vi "Adapt Experimental Data to Graph Entry.vi"(1 "Experiment Data":T1, 2 "Load Path":path) -> (0 "Populated Entry":T2)   [LabVIEW 2013]
uses:
  Serialization/Experiment/1.0.0/Types/Experiment Data.ctl
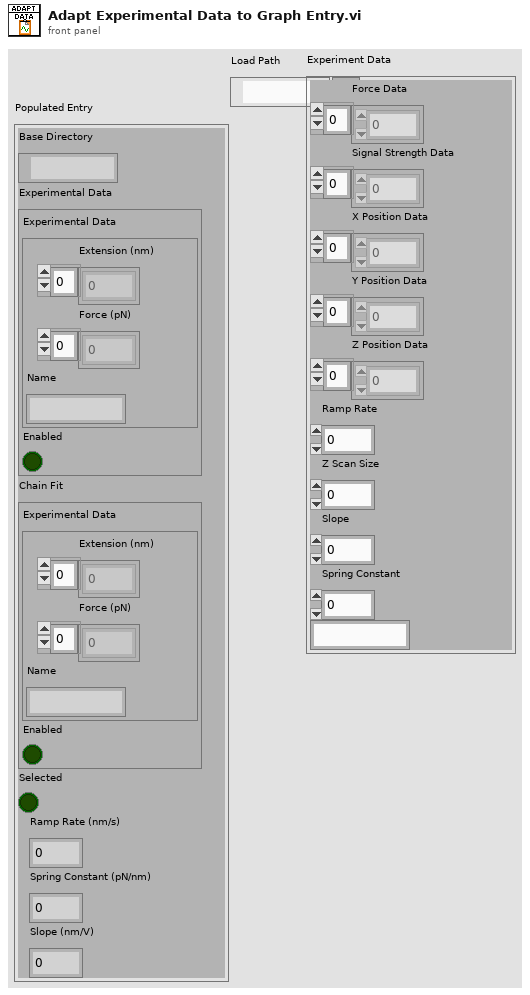
[diagram p1: front panel]
types:
  T1 = typedef "Experiment Data.ctl" = cluster{"Force Data":dbl[], "Signal Strength Data":dbl[], "X Position Data":dbl[], "Y Position Data":dbl[], "Z Position Data":dbl[], "Ramp Rate":dbl, "Z Scan Size":dbl, "Slope":dbl, "Spring Constant":dbl, "Version":string}
  T2 = cluster{"Base Directory":path, "Experimental Data":cluster{"Experimental Data":cluster{"Extension (nm)":dbl[], "Force (pN)":dbl[], "Name":string}, "Enabled":bool}, "Chain Fit":cluster{"Experimental Data":cluster{"Extension (nm)":dbl[], "Force (pN)":dbl[], "Name":string}, "Enabled":bool}, "Selected":bool, "Ramp Rate (nm/s)":dbl, "Spring Constant (pN/nm)":dbl, "Slope (nm/V)":dbl}
  T3 = cluster{"Extension (nm)":dbl[], "Force (pN)":dbl[], "Name":string}
  T4 = cluster{"Experimental Data":cluster{"Extension (nm)":dbl[], "Force (pN)":dbl[], "Name":string}, "Enabled":bool}
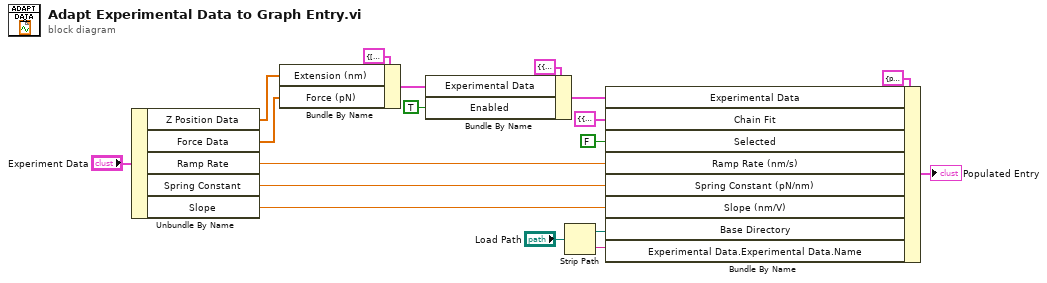
[diagram p0: block diagram]
diagram:
  n1 = Unbundle By Name("Experiment Data") -> ("Z Position Data"=w17:dbl[], "Force Data"=w16:dbl[], "Ramp Rate"=w12:dbl, "Spring Constant"=w11:dbl, "Slope"=w10:dbl)
  n2 = Bundle By Name(cluster=T3 {"Extension (nm)"=[], "Force (pN)"=[], "Name"=""} ("Experimental Data"), "Extension (nm)"=w17, "Force (pN)"=w16) -> (w7:T3)
  n3 = Bundle By Name(cluster=T4 {"Experimental Data"={"Extension (nm)"=[], "Force (pN)"=[], "Name"=""}, "Enabled"=FALSE} ("Experimental Data"), "Experimental Data"=w7, "Enabled"=TRUE) -> (w15:T4)
  n4 = Strip Path(path="Load Path") -> (stripped path=w4:path, name=w3:string)
  n5 = Bundle By Name(cluster=T2 {"Base Directory"=path "", "Experimental Data"={"Experimental Data"={"Extension (nm)"=[], "Force (pN)"=[], "Name"=""}, "Enabled"=FALSE}, "Chain Fit"={"Experimental Data"={"Extension (nm)"=[], "Force (pN)"=[], "Name"=""}, "Enabled"=FALSE}, "Selected"=FALSE, "Ramp Rate (nm/s)"=0.0, "Spring Constant (pN/nm)"=0.0, "Slope (nm/V)"=0.0} ("Graph Entry"), "Experimental Data"=w15, "Chain Fit"=T4 {"Experimental Data"={"Extension (nm)"=[], "Force (pN)"=[], "Name"=""}, "Enabled"=FALSE} ("Experimental Data"), "Selected"=FALSE, "Ramp Rate (nm/s)"=w12, "Spring Constant (pN/nm)"=w11, "Slope (nm/V)"=w10, "Base Directory"=w4, "Experimental Data.Experimental Data.Name"=w3) -> (→"Populated Entry":T2)
